vi "SelectMenu.vi"(0 "XRef":T24, 1 "Tag":T20, 2 "Point":T22, 3 "Click Type":T21, 4 "State In":T1={"BlockNodeState"={"Terminal Data"=[], "Instance Name"="", "Type Name"="", "Draw Style"=0, "Connector Pane Pattern"=0, "Flags"=0, "Grown Terminal List Order"=[], "Image"={"image type"=0, "image depth"=0, "image"=[], "mask"=[], "colors"=[], "Rectangle"={"left"=0, "top"=0, "right"=0, "bottom"=0}}}, "stateInfo"={"Data storage parameters"={"Name"="", "Format"="TDM", "Connection string"="", "use default"=TRUE}, "Object type"="root", "Selected properties"=[], "Object definitions"=[], "Refnum input wired"=enum."<none>", "Parent object type"="", "Parent object child property"="", "Channel options"=enum."Replace values at index", "PendingCommand"=enum."<none>", "Node style"=enum."Classic", "Only child objects"=FALSE, "TermSpecs"=[], "objectTypeWired"="", "Dynamic format"=FALSE, "Overwrite options"=enum."open or create", "Parameters"=variant, "Format"="", "Node type"=enum."UPDATE", "ImplicitExplicit"=enum."explicit", "Channel type"=enum."Waveform", "Use object with same name"=FALSE, "Show channel terminal"=FALSE, "LabVIEW Version"="", "DataTerminals"=enum."Express", "Size to text"=FALSE, "selected nodes in"=[]}} {"BlockNodeState"."Draw Style" items=["FunctionBlock", "ExpressVI", "Variable", "Elemental I/O", "32x32 Icon", "FunctionBlockCompact"]; "BlockNodeState"."Terminal Data"."Terminal Flags" format="%.0b"}) -> (14 "Reply":T19, 15 "State Out":T1={"BlockNodeState"={"Terminal Data"=[], "Instance Name"="", "Type Name"="", "Draw Style"=0, "Connector Pane Pattern"=0, "Flags"=0, "Grown Terminal List Order"=[], "Image"={"image type"=0, "image depth"=0, "image"=[], "mask"=[], "colors"=[], "Rectangle"={"left"=0, "top"=0, "right"=0, "bottom"=0}}}, "stateInfo"={"Data storage parameters"={"Name"="", "Format"="TDM", "Connection string"="", "use default"=TRUE}, "Object type"="root", "Selected properties"=[], "Object definitions"=[], "Refnum input wired"=enum."<none>", "Parent object type"="", "Parent object child property"="", "Channel options"=enum."Replace values at index", "PendingCommand"=enum."<none>", "Node style"=enum."Classic", "Only child objects"=FALSE, "TermSpecs"=[], "objectTypeWired"="", "Dynamic format"=FALSE, "Overwrite options"=enum."open or create", "Parameters"=variant, "Format"="", "Node type"=enum."UPDATE", "ImplicitExplicit"=enum."explicit", "Channel type"=enum."Waveform", "Use object with same name"=FALSE, "Show channel terminal"=FALSE, "LabVIEW Version"="", "DataTerminals"=enum."Express", "Size to text"=FALSE, "selected nodes in"=[]}} {"BlockNodeState"."Draw Style" items=["FunctionBlock", "ExpressVI", "Variable", "Elemental I/O", "32x32 Icon", "FunctionBlockCompact"]; "BlockNodeState"."Terminal Data"."Terminal Flags" format="%.0b"})   [LabVIEW 2017, in "Open Data Storage.xnode"]
uses:
  <vilib>/Platform/storage/lvStorage.llb/xStorage/Open Data Storage/Open Data Storage.xnode
  <vilib>/XNodeSupport/XNodeXNodeRef.ctl
  <vilib>/XNodeSupport/XNodeString.ctl
  <vilib>/XNodeSupport/XNodePoint.ctl
  <vilib>/XNodeSupport/XNodeInt.ctl
  <vilib>/XNodeSupport/XNodeClickTypes.ctl
  <vilib>/Platform/storage/lvStorage.llb/xStorage/Open Data Storage/State.ctl
  <vilib>/BlockNodeSupport/BlockNodeState.ctl
  <vilib>/BlockNodeSupport/TerminalData.ctl
  <vilib>/picture/picture.llb/imagedata.ctl
  <vilib>/Platform/storage/lvStorage.llb/dataStorageParams.ctl
  <vilib>/Platform/storage/lvStorage.llb/_selectedProp.ctl
  <vilib>/Platform/storage/lvStorage.llb/dataModel.ctl
  <vilib>/Platform/storage/Storage.llb/usiTypeDef.ctl
  <vilib>/Platform/storage/Storage.llb/usiPropDef.ctl
  <vilib>/express/express shared/ex_EditUserDefinedProperties/usiDataType.ctl
  <vilib>/Platform/storage/Storage.llb/specialProperties.ctl
  <vilib>/Platform/storage/Storage.llb/usiOverwriteOptions.ctl
  <vilib>/Platform/storage/lvStorage.llb/TerminalDef.ctl
  <vilib>/Platform/storage/lvStorage.llb/_TerminalStyle.ctl
  <vilib>/Utility/XNodeSupport.llb/XRect32.ctl
  <vilib>/Platform/storage/Storage.llb/usiSequenceRepresentation.ctl
  <vilib>/Platform/storage/lvStorage.llb/channelType.ctl
  <vilib>/Platform/storage/lvStorage.llb/_dataTerminals.ctl
  <vilib>/XNodeSupport/XNodeStringArray.ctl
  <vilib>/XNodeSupport/NI_XNodeSupport.lvlib
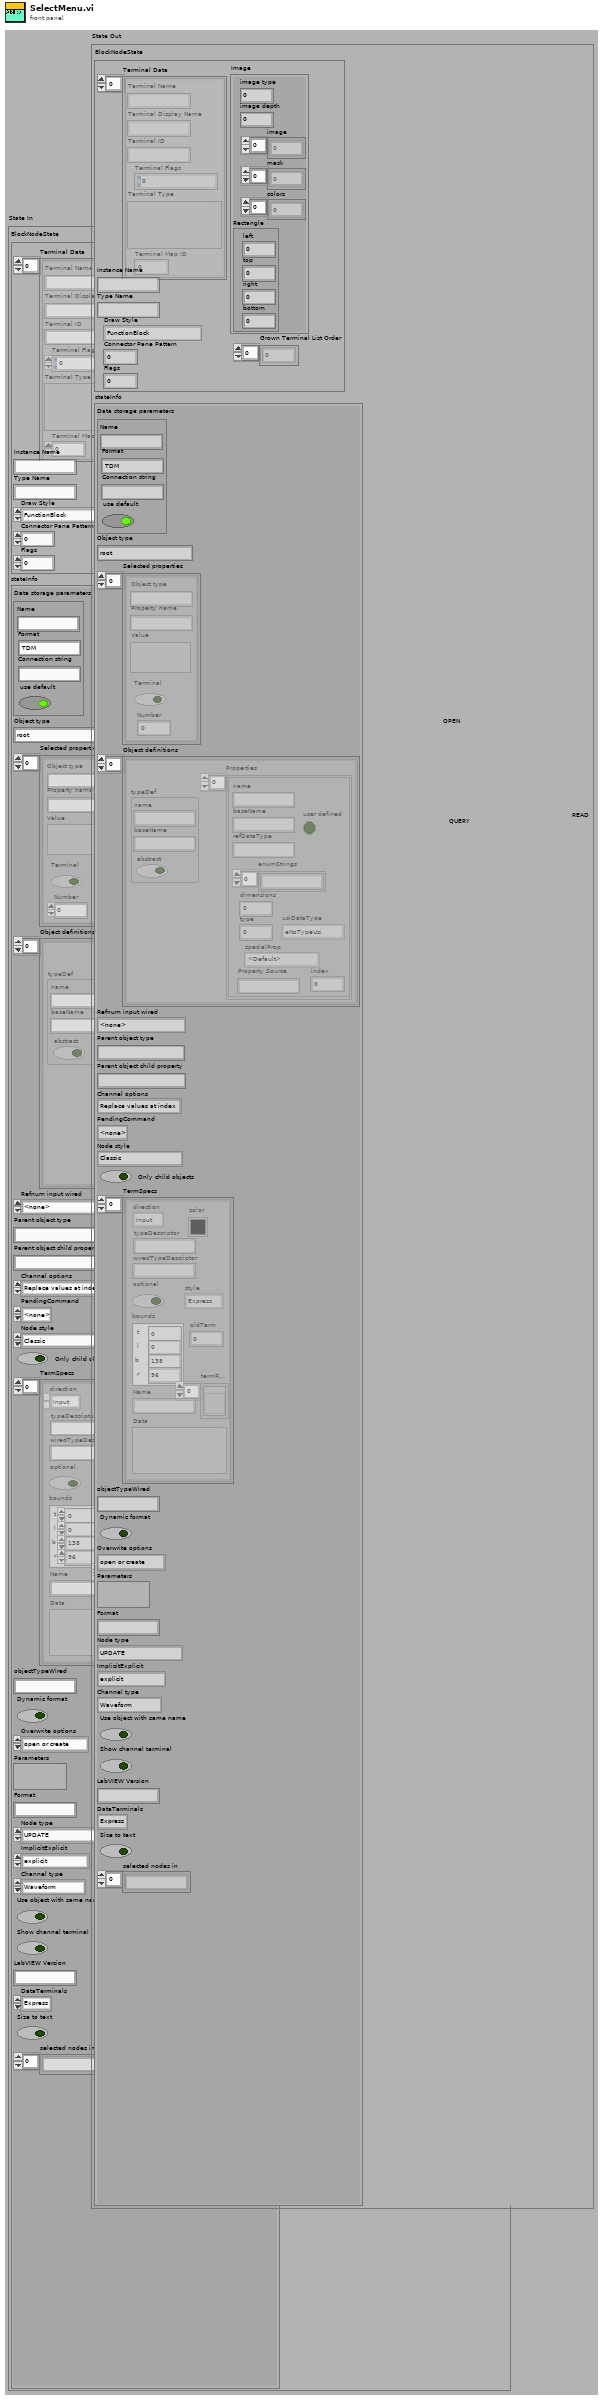
[diagram p1: front panel]
types:
  T1 = typedef "Open Data Storage.xnode/State.ctl" = cluster{"BlockNodeState":T2, "stateInfo":cluster{"Data storage parameters":T5, "Object type":string, "Selected properties":T6[], "Object definitions":T7[], "Refnum input wired":enum16{"Storage", "Generic object", "Typed object", "<none>"}, "Parent object type":string, "Parent object child property":string, "Channel options":T12, "PendingCommand":enum16{"<none>", "SelPopUp", "Init"}, "Node style":enum16{"Classic", "Express"}, "Only child objects":bool, "TermSpecs":T13[], "objectTypeWired":string, "Dynamic format":bool, "Overwrite options":enum16{"open", "open or create", "create or replace", "create", "open (read only)"}, "Parameters":variant, "Format":string, "Node type":enum16{"UPDATE", "READ", "QUERY", "CREATE CHILD", "CREATE", "CONNECT", "DISCONNECT"}, "ImplicitExplicit":T16, "Channel type":T17, "Use object with same name":bool, "Show channel terminal":bool, "LabVIEW Version":string, "DataTerminals":T18, "Size to text":bool, "selected nodes in":string[]}}
  T2 = typedef "BlockNodeState.ctl" = cluster{"Terminal Data":T3[], "Instance Name":string, "Type Name":string, "Draw Style":i32, "Connector Pane Pattern":i32, "Flags":i32, "Grown Terminal List Order":i32[], "Image":T4}
  T3 = typedef "TerminalData.ctl" = cluster{"Terminal Name":string, "Terminal Display Name":string, "Terminal ID":string, "Terminal Flags":i32, "Terminal Type":variant, "Terminal Map ID":i32}
  T4 = typedef "imagedata.ctl" = cluster{"image type":i32, "image depth":i32, "image":u8[], "mask":u8[], "colors":u32[], "Rectangle":cluster{"left":i16, "top":i16, "right":i16, "bottom":i16}}
  T5 = typedef "dataStorageParams.ctl" = cluster{"Name":string, "Format":string, "Connection string":string, "use default":bool}
  T6 = typedef "_selectedProp.ctl" = cluster{"Object type":string, "Property name":string, "Value":variant, "Terminal":bool, "Number":i32}
  T7 = typedef "dataModel.ctl" = cluster{"typeDef":T8, "Properties":T9[]}
  T8 = typedef "usiTypeDef.ctl" = cluster{"name":string, "baseName":string, "abstract":bool}
  T9 = typedef "usiPropDef.ctl" = cluster{"name":string, "baseName":string, "refDataType":string, "dimensions":i32, "type":i32, "user defined":bool, "enumStrings":string[], "usiDataType":T10, "specialProp":T11, "Property Source":string, "index":i32}
  T10 = typedef "usiDataType.ctl" = enum16{"eNoTypeUsi", "eInt8Usi", "eInt16Usi", "eInt32Usi", "eInt64Usi", "eUInt8Usi", "eUInt16Usi", "eUInt32Usi", "eUInt64Usi", "eFloat32Usi", "eFloat64Usi", "- 0", "- 1", "- 2", "- 3", "- 4", "- 5", "- 6", "- 7", "- 8", "- 9", "eString8Usi", "eString16Usi", "eStringUsi", "eEnumUsi", "- 10", "- 11", "- 12", "- 13", "- 14", "eTimeUsi", "- 15", "- 16", "- 17", "- 18", "- 19", "- 20", "- 21", "- 22", "- 23", "eInstanceUsi", "eStoreUsi"}
  T11 = typedef "specialProperties.ctl" = enum16{"<Default>", "Channel Values", "AppendReplace", "ChannelFlags", "ValueFlags", "ImplicitExplicit", "InsertIndex", "ValuesCount", "ComparisonOperator", "Cluster", "DAQmx Channel"}
  T12 = typedef "usiOverwriteOptions.ctl" = enum16{"Append values", "Replace values at index", "Replace all values", "Append if timeline aligns"}
  T13 = typedef "TerminalDef.ctl" = cluster{"direction":enum16{"Input", "Output"}, "typeDescriptor":string, "color":u32, "oldTerm":i32, "style":T14, "optional":bool, "bounds":T15, "termRefs":refnum<vi>[], "Name":string, "Data":variant, "wiredTypeDescriptor":string}
  T14 = typedef "_TerminalStyle.ctl" = enum16{"Express", "Collapsed", "Internal"}
  T15 = typedef "XRect32.ctl" = cluster{"t":i32, "l":i32, "b":i32, "r":i32}
  T16 = typedef "usiSequenceRepresentation.ctl" = enum16{"explicit", "implicit"}
  T17 = typedef "channelType.ctl" = enum16{"Waveform", "Array of Double", "Array of String", "DDT", "Array of UInt8", "Array of Int16", "Array of Int32", "Array of Single", "Array of DateTime", "Array of Waveform", "none", "DateTime", "String", "Double", "Single", "UInt8", "Int16", "Int32"}
  T18 = typedef "_dataTerminals.ctl" = enum16{"Express", "Cluster"}
  T19 = typedef "NI_XNodeSupport.lvlib/XNodeStringArray.ctl" = T20[]
  T20 = typedef "NI_XNodeSupport.lvlib/XNodeString.ctl" = string
  T21 = typedef "NI_XNodeSupport.lvlib/XNodeClickTypes.ctl" = enum32{"Operate Click", "Popup Click"}
  T22 = typedef "NI_XNodeSupport.lvlib/XNodePoint.ctl" = cluster{"H":T23, "V":T23}
  T23 = typedef "NI_XNodeSupport.lvlib/XNodeInt.ctl" = i32
  T24 = typedef "NI_XNodeSupport.lvlib/XNodeXNodeRef.ctl" = refnum<vi>
  T25 = cluster{"Data storage parameters":T5, "Object type":string, "Selected properties":T6[], "Object definitions":T7[], "Refnum input wired":enum16{"Storage", "Generic object", "Typed object", "<none>"}, "Parent object type":string, "Parent object child property":string, "Channel options":T12, "PendingCommand":enum16{"<none>", "SelPopUp", "Init"}, "Node style":enum16{"Classic", "Express"}, "Only child objects":bool, "TermSpecs":T13[], "objectTypeWired":string, "Dynamic format":bool, "Overwrite options":enum16{"open", "open or create", "create or replace", "create", "open (read only)"}, "Parameters":variant, "Format":string, "Node type":enum16{"UPDATE", "READ", "QUERY", "CREATE CHILD", "CREATE", "CONNECT", "DISCONNECT"}, "ImplicitExplicit":T16, "Channel type":T17, "Use object with same name":bool, "Show channel terminal":bool, "LabVIEW Version":string, "DataTerminals":T18, "Size to text":bool, "selected nodes in":string[]}
  T26 = typedef "_stateInfoWriteProps.ctl" = cluster{"Data storage parameters":T5, "Object type":string, "Selected properties":T6[], "Object definitions":T7[], "Refnum input wired":enum16{"Storage", "Generic object", "Typed object", "<none>"}, "Parent object type":string, "Parent object child property":string, "Channel options":T12, "PendingCommand":enum16{"<none>", "SelPopUp", "Init"}, "Node style":enum16{"Classic", "Express"}, "Only child objects":bool, "TermSpecs":T13[], "objectTypeWired":string, "Dynamic format":bool, "Overwrite options":enum16{"open", "open or create", "create or replace", "create", "open (read only)"}, "Parameters":variant, "Format":string, "Node type":enum16{"UPDATE", "READ", "QUERY", "CREATE CHILD", "CREATE", "CONNECT", "DISCONNECT"}, "ImplicitExplicit":T16, "Channel type":T17, "Use object with same name":bool, "Show channel terminal":bool, "LabVIEW Version":string, "DataTerminals":T18, "Size to text":bool, "selected nodes in":string[]}
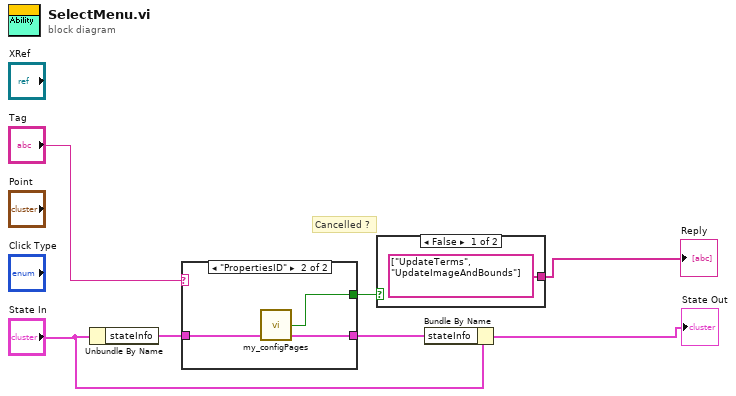
[diagram p0: block diagram]
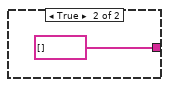
[diagram p2: hidden frame]
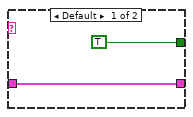
[diagram p3: hidden frame]
diagram:
  # "Cancelled ?"
  n1 = Unbundle By Name("State In") -> ("stateInfo"=w7:T25)
  n2 = case shown="\"PropertiesID\"" "Tag" {
    tunnel: w7 -> [w9 w12]
    tunnel: [w9 w11] -> w6
    tunnel: [TRUE w10] -> w5
    frame Default {
    }
    frame "PropertiesID" {
      n3 = call <vilib>:"my_configPages.vi"("stateInfo in"=w12) -> ("stateInfo out"=w11:T26, "Cancelled"=w10:bool)  [unwired: 3 in]
    }
  }
  n4 = case shown="False" w5 {
    tunnel: [T19 ["UpdateTerms", "UpdateImageAndBounds"] ("Reply") T19 [] ("Reply")] -> w4
    frame False {
    }
    frame True {
    }
  }
  "Reply" <- w4
  n5 = Bundle By Name(cluster="State In", "stateInfo"=w6) -> (→"State Out":T1)
